vi "New Task Request.vi"(8 "error in (no error)":errorcluster, 10 "Task":variant, 11 "BuildWorker in":refnum<class "BuildWorker.lvclass">) -> (0 "error out":errorcluster, 3 "BuildWorker out":refnum<class "BuildWorker.lvclass">)   [LabVIEW 2017, in "BuildWorker.lvlib" / "BuildWorker.lvclass"]
uses:
  BuildWorker.lvclass
  Classes/Task/Task.lvclass
  Classes/Task/Status.ctl
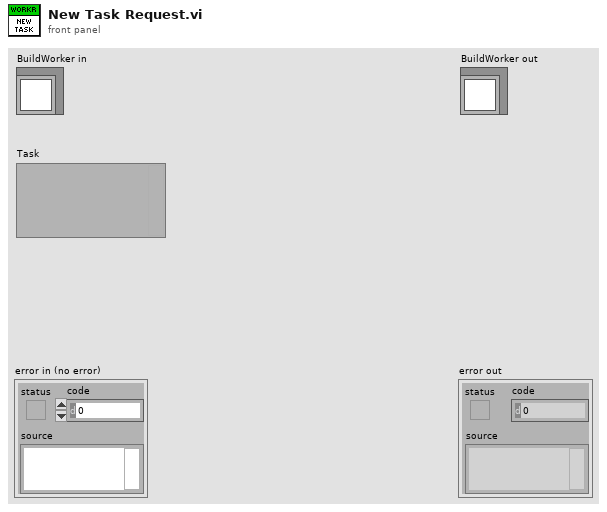
[diagram p1: front panel]
types:
  T1 = typedef "Task Interface.lvlib/Task.lvclass/Status.ctl" = enum16{"Created", "Added", "Pending", "Queued", "Processing", "Cleaning", "Building", "Finished", "Failed", "Removed", "Not found"}
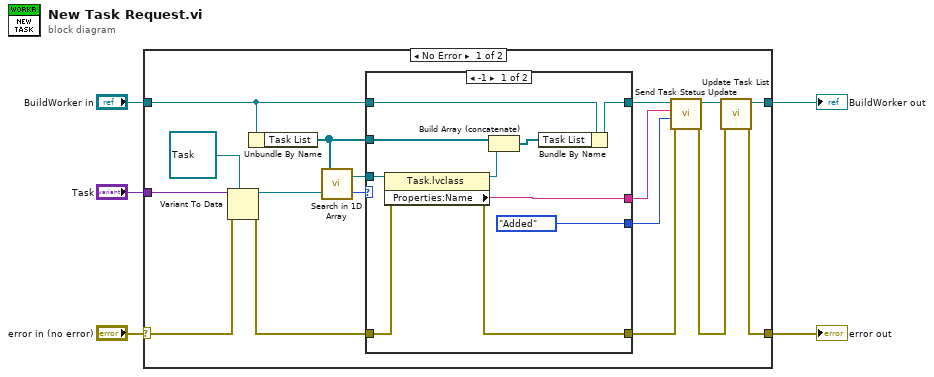
[diagram p0: block diagram]
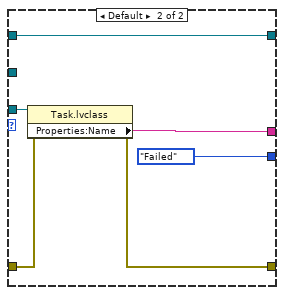
[diagram p2: hidden frame]
diagram:
  n1 = case shown="No Error" "error in (no error)" {
    selector: "error in (no error)" -> [w20 w40]
    tunnel: [w16 w40] -> w4
    tunnel: [w17 w39] -> w2
    tunnel: "BuildWorker in" -> [w19 w39]
    tunnel: "Task" -> [w22 _]
    frame No Error {
      n2 = Variant To Data(error in=w20, type=refnum<class "Task.lvclass"> refnum ("Task.lvclass"), Variant=w22) -> (data=w9:refnum<class "Task.lvclass">, error out=w18:errorcluster)
      n3 = Unbundle By Name(w19) -> ("Task List"=w10:refnum<class "Task.lvclass">[])
      n4 = call "Search in 1D Array.vi"("Task in"=w9, "Task Array"=w10) -> ("index of element"=w7:i32, "Task"=w8:refnum<class "Task.lvclass">)
      n5 = case shown="-1" w7 {
        tunnel: w19 -> [w32 w38]
        tunnel: w18 -> [w29 w35]
        tunnel: [w28 w38] -> w15
        tunnel: [w27 w34] -> w13
        tunnel: [w26 w36] -> w11
        tunnel: [Status."Added" ("Status") Status."Failed" ("Status")] -> w6
        tunnel: w10 -> [w25 _]
        tunnel: w8 -> [w24 w37]
        frame -1 {
          n6 = property class="Task.lvclass"(reference=w24, error in=w29) -> (reference out=w30:refnum<class "Task.lvclass">, error out=w27:errorcluster, "Properties:Name"=w26:string)
          n7 = Build Array (concatenate)(w25, w30) -> (w31:refnum<class "Task.lvclass">[])
          n8 = Bundle By Name(cluster=w32, "Task List"=w31) -> (w28:refnum<class "BuildWorker.lvclass">)
        }
        frame Default {
          n9 = property class="Task.lvclass"(reference=w37, error in=w35) -> (error out=w34:errorcluster, "Properties:Name"=w36:string)  [unwired: 1 out]
        }
      }
      n10 = call "Send Task Status Update.vi"("error in (no error)"=w13, "Status"=w6, "Task Name"=w11, "BuildWorker in"=w15) -> ("error out"=w12:errorcluster, "BuildWorker out"=w14:refnum<class "BuildWorker.lvclass">)  [unwired: 6 in]
      n11 = call "Update Task List.vi"("error in (no error)"=w12, "BuildWorker in"=w14) -> ("error out"=w16:errorcluster, "BuildWorker out"=w17:refnum<class "BuildWorker.lvclass">)  [unwired: 8 in]
    }
    frame Error {
    }
  }
  "error out" <- w4
  "BuildWorker out" <- w2
